vi "3-D Rotation using 3-points.vi"(4 "Present Position":T1 {"Point3" format="%.2f"; "Point2" format="%.2f"; "Point1" format="%.2f"}, 6 "Initial Position":T1 {"Point3" format="%.2f"; "Point2" format="%.2f"; "Point1" format="%.2f"}, 7 "Radius of eyeball in pixels":dbl=240.0 format="%.2f") -> (0 "T":dbl=9.000000000000245 format="%.2f", 1 "V":dbl=-19.000000000000494 format="%.2f", 2 "H":dbl=7.999999999999464 format="%.2f", 3 "Valid Calculation":bool)   [LabVIEW 2013, in "3 dot tracker.lvlib"]
uses:
  3 dot tracker.lvlib
  <vilib>/Analysis/baseanly.llb/Real A x B.vi
  <vilib>/Analysis/_algsub.llb/Real PseudoInverse Matrix.vi
  comm/fick-matrix/fick-matrix.lvlib
  <vilib>/Analysis/NI_AALBase.lvlib
  <vilib>/Analysis/NI_AALPro.lvlib
panel:
  # "3D eye orientation given three points"
  # "Dr. A. Migliaccio 6-19-03"
  # "Fick Angles"
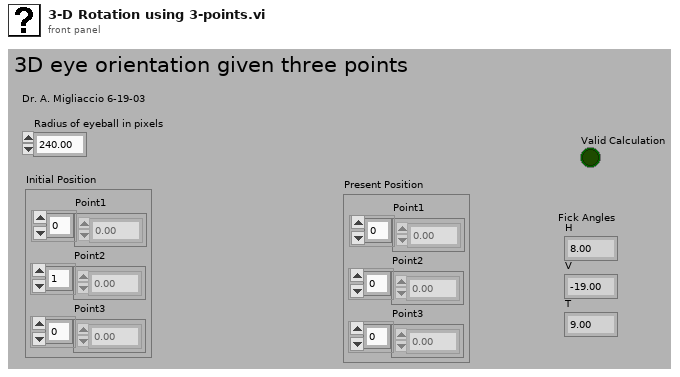
[diagram p1: front panel]
types:
  T1 = cluster{"Point1":dbl[], "Point2":dbl[], "Point3":dbl[]}
  T2 = typedef "NI_Matrix.lvlib/RealMatrix.ctl" = dbl[][]
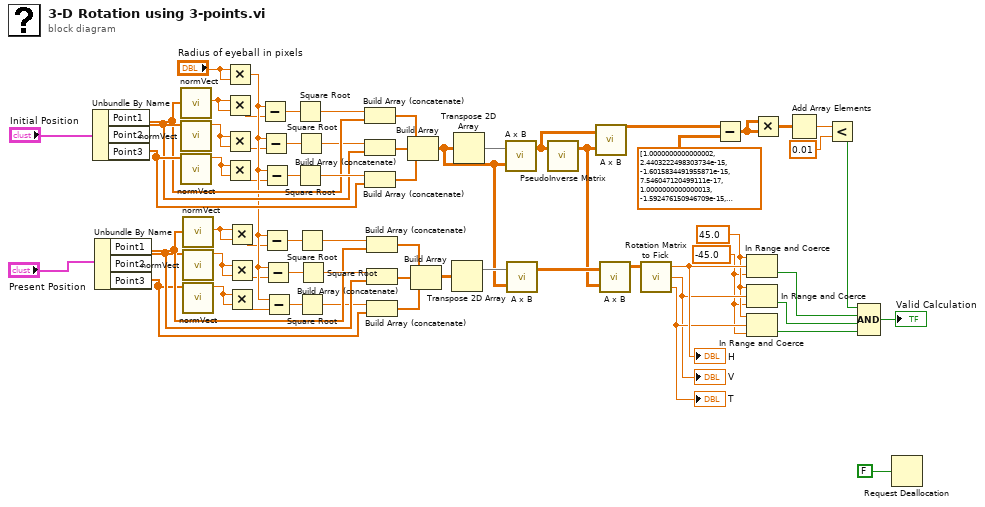
[diagram p0: block diagram]
diagram:
  w7 = -45.0 ("upper limit")
  w8 = 45.0 ("upper limit")
  n1 = Unbundle By Name("Initial Position") -> ("Point1"=w49:dbl[], "Point2"=w50:dbl[], "Point3"=w52:dbl[])
  n2 = Unbundle By Name("Present Position") -> ("Point1"=w44:dbl[], "Point2"=w43:dbl[], "Point3"=w41:dbl[])
  n3 = call "normVect.vi"("Array"=w49) -> ("norm"=w58:dbl)  [unwired: 10 in]
  n4 = call "normVect.vi"("Array"=w50) -> ("norm"=w57:dbl)  [unwired: 10 in]
  n5 = call "normVect.vi"("Array"=w52) -> ("norm"=w56:dbl)  [unwired: 10 in]
  n6 = call "normVect.vi"("Array"=w44) -> ("norm"=w35:dbl)  [unwired: 10 in]
  n7 = call "normVect.vi"("Array"=w43) -> ("norm"=w36:dbl)  [unwired: 10 in]
  n8 = call "normVect.vi"("Array"=w41) -> ("norm"=w37:dbl)  [unwired: 10 in]
  n9 = Multiply(x="Radius of eyeball in pixels", y="Radius of eyeball in pixels") -> (x*y=w19:dbl)
  n10 = Multiply(x=w58, y=w58) -> (x*y=w13:dbl)
  n11 = Multiply(x=w57, y=w57) -> (x*y=w14:dbl)
  n12 = Multiply(x=w56, y=w56) -> (x*y=w15:dbl)
  n13 = Multiply(x=w35, y=w35) -> (x*y=w16:dbl)
  n14 = Multiply(x=w36, y=w36) -> (x*y=w17:dbl)
  n15 = Multiply(x=w37, y=w37) -> (x*y=w18:dbl)
  n16 = Subtract(x=w19, y=w13) -> (x-y=w55:dbl)
  n17 = Subtract(x=w19, y=w14) -> (x-y=w54:dbl)
  n18 = Subtract(x=w19, y=w15) -> (x-y=w53:dbl)
  n19 = Subtract(x=w19, y=w16) -> (x-y=w38:dbl)
  n20 = Subtract(x=w19, y=w17) -> (x-y=w39:dbl)
  n21 = Subtract(x=w19, y=w18) -> (x-y=w40:dbl)
  n22 = Square Root(x=w55) -> (sqrt(x)=w47:dbl)
  n23 = Square Root(x=w53) -> (sqrt(x)=w51:dbl)
  n24 = Square Root(x=w54) -> (sqrt(x)=w48:dbl)
  n25 = Square Root(x=w38) -> (sqrt(x)=w46:dbl)
  n26 = Square Root(x=w40) -> (sqrt(x)=w42:dbl)
  n27 = Square Root(x=w39) -> (sqrt(x)=w45:dbl)
  n28 = Build Array (concatenate)(w47, w49) -> (w34:dbl[])
  n29 = Build Array (concatenate)(w48, w50) -> (w33:dbl[])
  n30 = Build Array (concatenate)(w51, w52) -> (w32:dbl[])
  n31 = Build Array (concatenate)(w46, w44) -> (w31:dbl[])
  n32 = Build Array (concatenate)(w45, w43) -> (w30:dbl[])
  n33 = Build Array (concatenate)(w42, w41) -> (w29:dbl[])
  n34 = Build Array(w34, w33, w32) -> (w28:dbl[][])
  n35 = Build Array(w31, w30, w29) -> (w27:dbl[][])
  n36 = Transpose 2D Array(2D array=w27) -> (transposed array=w65:dbl[][])
  n37 = Transpose 2D Array(2D array=w28) -> (transposed array=w64:dbl[][])
  n38 = call-poly <vilib>:"A x B.vi"("B"=w28, "A"=w64) -> ("A x B"=w62:T2)  [unwired: 1 out]
  n39 = call-poly <vilib>:"A x B.vi"("B"=w28, "A"=w65) -> ("A x B"=w63:T2)  [unwired: 1 out]
  n40 = call-poly <vilib>:"PseudoInverse Matrix.vi"("Input Matrix"=w62) -> ("PseudoInverse Matrix"=w61:T2)  [unwired: 1 in, 1 out]
  n41 = call-poly <vilib>:"A x B.vi"("B"=w61, "A"=w62) -> ("A x B"=w25:T2)  [unwired: 1 out]
  n42 = call-poly <vilib>:"A x B.vi"("B"=w61, "A"=w63) -> ("A x B"=w26:T2)  [unwired: 1 out]
  n43 = call "Rotation Matrix to Fick.vi"("A"=w26) -> ("T"=w10:dbl, "V"=w9:dbl, "H"=w11:dbl)  [unwired: 2 in]
  "H" <- w11
  "V" <- w9
  "T" <- w10
  n44 = Subtract(x=w25, y=dbl[][] [[1.0000000000000002, 2.4403222498303734e-15, -1.6015834491955871e-15], [7.546047120499111e-17, 1.0000000000000013, -1.592476150946709e-15], [1.687018580387445e-16, 2.0660556598883772e-15, 0.9999999999999976]] ("Identity Matrix")) -> (x-y=w23:T2)
  n45 = In Range and Coerce(upper limit=w8, x=w11, lower limit=w7) -> (In Range?=w5:bool)  [unwired: 1 out]
  n46 = In Range and Coerce(upper limit=w8, x=w9, lower limit=w7) -> (In Range?=w4:bool)  [unwired: 1 out]
  n47 = In Range and Coerce(upper limit=w8, x=w10, lower limit=w7) -> (In Range?=w3:bool)  [unwired: 1 out]
  n48 = Multiply(x=w23, y=w23) -> (x*y=w22:T2)
  n49 = Add Array Elements(numeric array=w22) -> (sum=w21:dbl)
  n50 = Less?(x=w21, y=0.01) -> (x < y?=w6:bool)
  n51 = Compound Arithmetic op=AND(w6, w5, w4, w3) -> (→"Valid Calculation":bool)
  n52 = Request Deallocation(FALSE ("flag")) -> ()
